vi "CalcDiv.vi"(0 "Pixel size, um":dbl, 1 "Focus, mm":dbl, 5 "Threshold, %":dbl, 9 "Array":dbl[](array[numeric]), 11 "SAC/FAC":bool=TRUE, 12 "Numeric in":i32, 13 "new picture in":picture) -> (4 "Beam Params":T1, 10 "new picture out":picture)   [LabVIEW 2017]
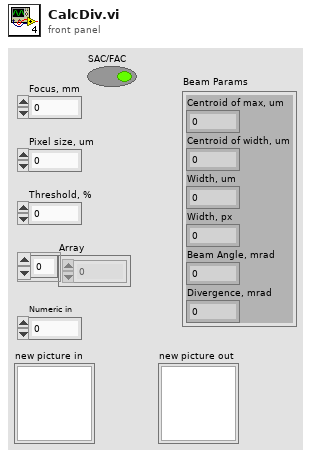
[diagram p1: front panel]
types:
  T1 = cluster{"Centroid of max, um":dbl, "Centroid of width, um":dbl, "Width, um":dbl, "Width, px":i32, "Beam Angle, mrad":dbl, "Divergence, mrad":dbl}
  T2 = cluster{dbl, dbl, "Width, um":dbl, i32, "Divergence, mrad":dbl, "Divergence, mrad":dbl}
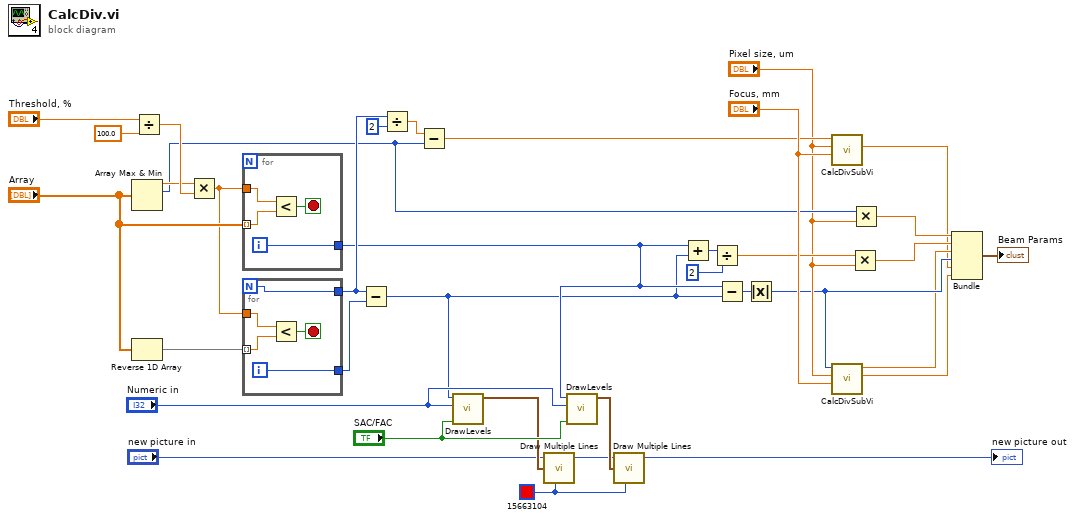
[diagram p0: block diagram]
diagram:
  w24 = u32 15663104 ("color(black)")
  n1 = Array Max & Min(array="Array") -> (max value=w29:dbl, max index (indices)=w10:i32)  [unwired: 2 out]
  n2 = Reverse 1D Array(array="Array") -> (reversed array=w20:dbl[])
  n3 = Divide(x="Threshold, %", y=100.0) -> (x/y=w30:dbl)
  n4 = Multiply(x=w29, y=w30) -> (x*y=w31:dbl)
  n5 = for {
    tunnel: w31 -> [w40]
    tunnel: "Array" -> [w37] mode=indexing
    tunnel: [w38] -> w14
    i -> [w38]
    stop <- w39 stop-if-true
    n6 = Less?(x=w40, y=w37) -> (x < y?=w39:bool)
  }
  n7 = for {
    N -> [w41]
    tunnel: w31 -> [w45]
    tunnel: w20 -> [w42] mode=indexing
    tunnel: [w43] -> w21
    tunnel: [w41] -> w18
    i -> [w43]
    stop <- w44 stop-if-true
    n8 = Less?(x=w45, y=w42) -> (x < y?=w44:bool)
  }
  n9 = Subtract(x=w18, y=w21) -> (x-y=w13:i32)
  n10 = Divide(x=w18, y=2) -> (x/y=w16:dbl)
  n11 = Subtract(x=w16, y=w10) -> (x-y=w15:dbl)
  n12 = call "DrawLevels.vi"("SAC/FAC"="SAC/FAC", "Size"="Numeric in", "Ind"=w13) -> ("Array"=w23:cluster{"theta (deg)":i32, i32}[])  [unwired: 8 in]
  n13 = call <vilib>:"Draw Multiple Lines.vi"("picture"="new picture in", "line endpoints"=w23, "color(black)"=w24) -> ("new picture"=w28:picture)  [unwired: 6 in]
  n14 = call "DrawLevels.vi"("SAC/FAC"="SAC/FAC", "Size"="Numeric in", "Ind"=w14) -> ("Array"=w33:cluster{"theta (deg)":i32, i32}[])  [unwired: 8 in]
  n15 = call <vilib>:"Draw Multiple Lines.vi"("picture"=w28, "line endpoints"=w33, "color(black)"=w24) -> ("new picture"=→"new picture out":picture)  [unwired: 6 in]
  n16 = Add(x=w14, y=w13) -> (x+y=w12:i32)
  n17 = Divide(x=w12, y=2) -> (x/y=w9:dbl)
  n18 = Subtract(x=w14, y=w13) -> (x-y=w32:i32)
  n19 = Absolute Value(x=w32) -> (abs(x)=w6:i32)
  n20 = call "CalcDivSubVi.vi"("Focus, mm"="Focus, mm", "Pixel size, um"="Pixel size, um", "Width, px"=w15) -> ("Divergence, mrad"=w1:dbl)  [unwired: 7 in, 1 out]
  n21 = call "CalcDivSubVi.vi"("Focus, mm"="Focus, mm", "Pixel size, um"="Pixel size, um", "Width, px"=w6) -> ("Divergence, mrad"=w2:dbl, "Width, um"=w5:dbl)  [unwired: 7 in]
  n22 = Multiply(x=w9, y="Pixel size, um") -> (x*y=w4:dbl)
  n23 = Multiply(x=w10, y="Pixel size, um") -> (x*y=w3:dbl)
  n24 = Bundle(w3, w4, "Width, um"=w5, w6, "Divergence, mrad"=w1, "Divergence, mrad"=w2) -> (→"Beam Params":T2)  [unwired: 1 in]
